vi "StepSize for Simloop.vi"() -> (2 "Numeric":dbl)   [LabVIEW 2020]
panel:
  out "Time per Iteration":u32
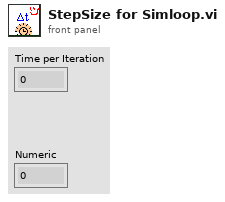
[diagram p1: front panel]
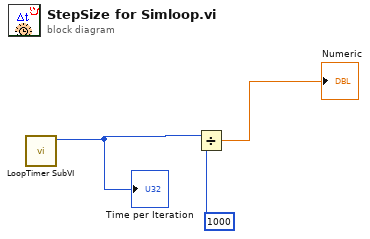
[diagram p0: block diagram]
diagram:
  n1 = call "LoopTimer SubVI.vi"() -> ("Numeric"=w1:u32)  [unwired: 11 in]
  "Time per Iteration" <- w1
  n2 = Divide(x=w1, y=u32 1000) -> (x/y=→"Numeric":dbl)
